vi "DecideFPS.vi"(8 "error in":errorcluster, 9 "分辨率":u16(ring) items=["640*512"], 10 "分辨率索引":i32[](array[numeric]), 11 "camera_stream_info[]":T1(array[cluster])) -> (0 "error out":errorcluster, 1 "fps":u16(ring) items=["30", "25", ""], 2 "fpsalll":u32[](array[numeric]))   [LabVIEW 2016]
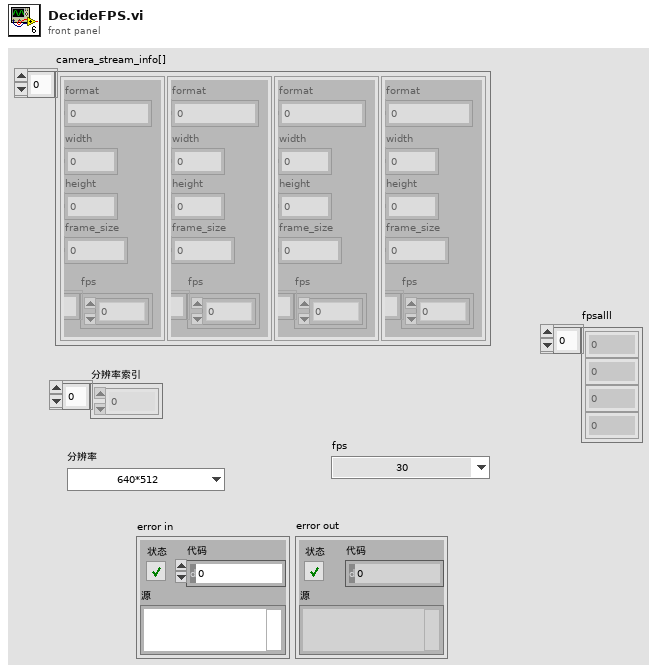
[diagram p1: front panel]
types:
  T1 = cluster{"format":u64, "width":u32, "height":u32, "frame_size":u32, "fps":u32[]}[]
  T2 = cluster{"format":u64, "width":u32, "height":u32, "frame_size":u32, "fps":u32[]}
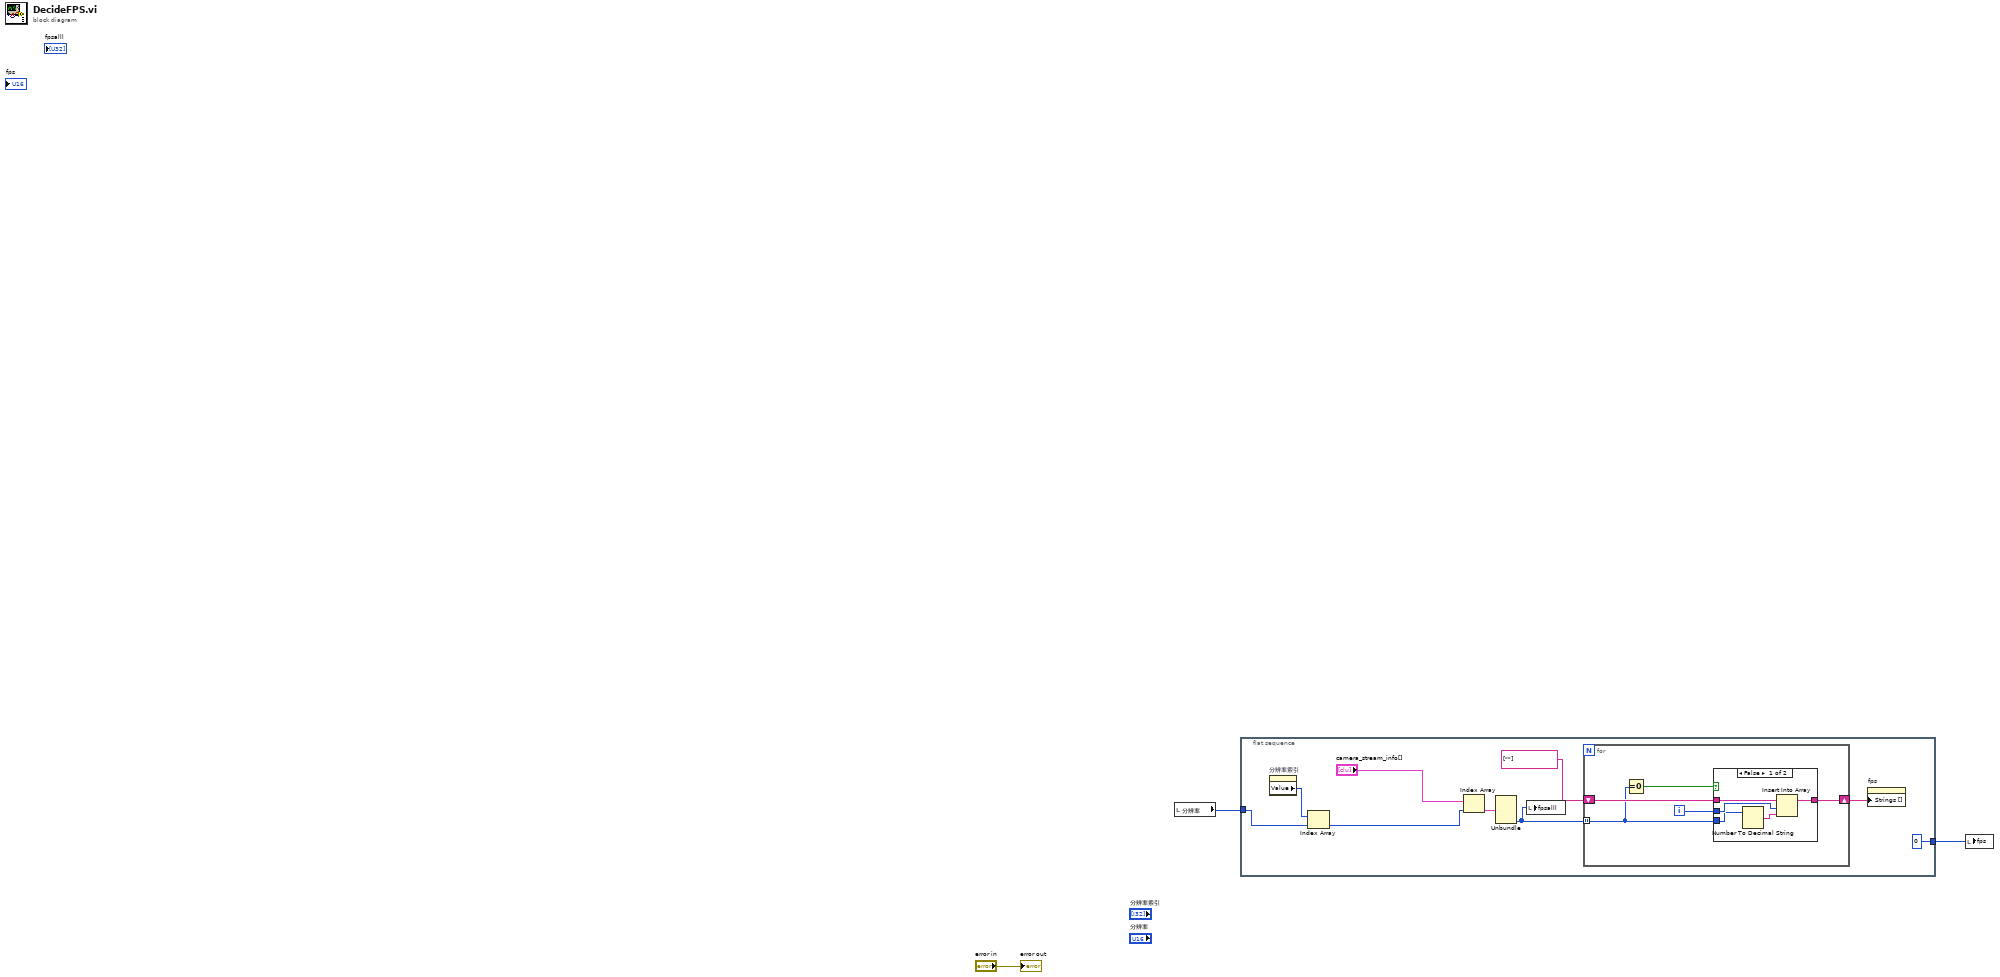
[diagram p0: block diagram]
diagram:
  n1 = local read "分辨率"() -> (w3:u16)
  n2 = flat-sequence {
    tunnel: w3 -> [w6]
    tunnel: [u16 0] -> w2
    frame #0 {
      n3 = property on="分辨率索引" class="Arr (strict)"() -> ("Value"=w7:i32[])  [unwired: 2 in, 2 out]
      n4 = Index Array(array=w7, index=w6) -> (element=w5:i32)
      n5 = Index Array(array="camera_stream_info[]", index=w5) -> (element=w10:T2)
      n6 = Unbundle(w10) -> ("fps"=w9:u32[])  [unwired: 4 out]
      n7 = local write "fpsalll"(w9) -> ()
      n8 = for {
        shift-right: [w16] -> w11
        shift-left: string[] [""] -> [w17]
        tunnel: w9 -> [w14] mode=indexing
        i -> [w13]
        n9 = Equal To 0?(x=w14) -> (x = 0?=w15:bool)
        n10 = case shown="False" w15 {
          tunnel: w13 -> [w22 _]
          tunnel: w17 -> [w21 w23]
          tunnel: [w19 w23] -> w16
          tunnel: w14 -> [w18 _]
          frame False {
            n11 = Number To Decimal String(number=w18) -> (decimal integer string=w20:string)  [unwired: 1 in]
            n12 = Insert Into Array(array=w21, index=w22, new element=w20) -> (w19:string[])
          }
          frame True {
          }
        }
      }
      n13 = property on="fps" class="Ring (strict)"("Strings []"=w11) -> ()  [unwired: 2 in, 2 out]
    }
  }
  n14 = local write "fps"(w2) -> ()
  "error out" <- "error in"
